vi "CC Next ID.vi"(8 "error in (no error)":errorcluster) -> (0 "error out":errorcluster, 2 "BlockID string":string, 3 "BlockID":i32)   [LabVIEW 2021]
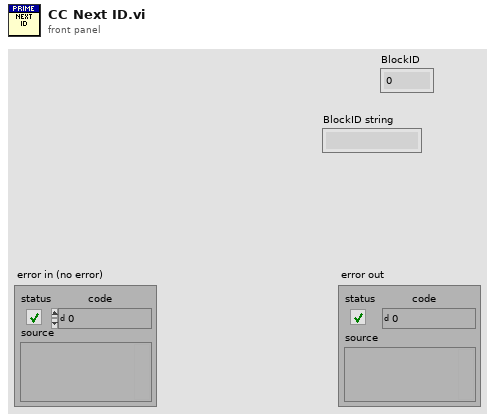
[diagram p1: front panel]
types:
  T1 = typedef "CC cluster BlockID.ctl" = cluster{"BlockID":i32}
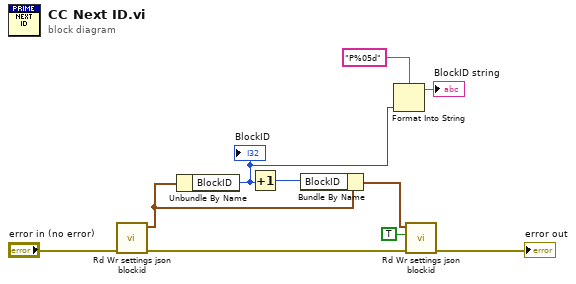
[diagram p0: block diagram]
diagram:
  n1 = call "Rd Wr settings json blockid.vi"("error in (no error)"="error in (no error)") -> ("error out"=w6:errorcluster, "Block ID"=w9:T1)  [unwired: 9 in]
  n2 = Unbundle By Name(w9) -> ("BlockID"=w2:i32)
  "BlockID" <- w2
  n3 = Increment(x=w2) -> (x+1=w8:i32)
  n4 = Bundle By Name(cluster=w9, "BlockID"=w8) -> (w7:T1)
  n5 = Format Into String(format string="P%05d", w2) -> (resulting string=→"BlockID string":string)  [unwired: 2 in, 1 out]
  n6 = call "Rd Wr settings json blockid.vi"("error in (no error)"=w6, "Write? (F:Read)"=TRUE, "Block ID"=w7) -> ("error out"=→"error out":errorcluster)  [unwired: 7 in, 1 out]
